vi "E441X_PM_Get_Sensor_Type.vi"(0 "VISA session":refnum<visa-resource-name>, 5 "Channel (0: A)":i32(ring) items=["A", "B"], 11 "error in (no error)":errorcluster {"code" format="%.0x"}) -> (4 "dup VISA session":refnum<visa-resource-name>, 6 "State":bool=TRUE, 10 "Sensor Type":string, 15 "error out":errorcluster {"code" format="%.0x"})   [LabVIEW 2015]
doc: "This VI returns the type of sensor connected to the selected input."
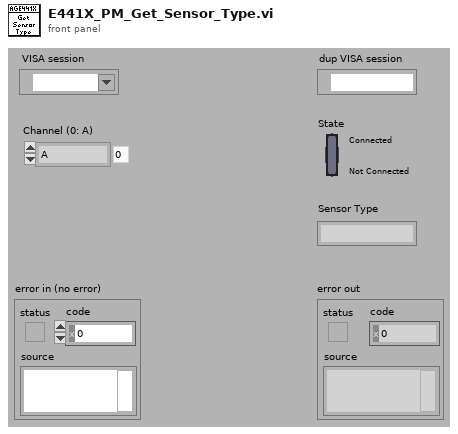
[diagram p1: front panel]
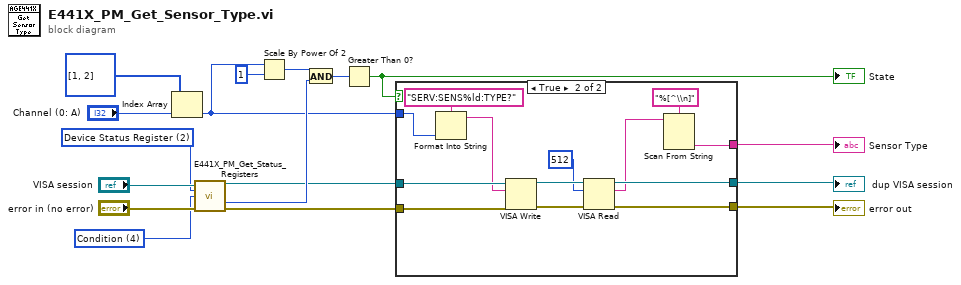
[diagram p0: block diagram]
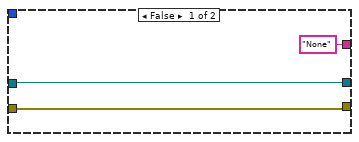
[diagram p2: hidden frame]
diagram:
  w14 = 4 items=["Enable"=2, "Negative Transition"=0, "Positive Transition"=1, "Event"=3, "Condition"=4] ("Register Part (2: Enable)")
  w15 = 2 items=["Service Request Enable Register (SRE)", "Standard Event Status Enable Register (ESE)", "Device Status Register", "Operation Status Register", "Questionable Status Register", "Operation Status Calibration", "Operation Status Measuring", "Operation Status Trigger", "Operation Status Sense", "Operation Status Low Limit Fail", "Operation Status Upper Limit Fail", "Questionable Status Power", "Questionable Status Calibration"] ("Register (4: Questionable Status Register)")
  n1 = Index Array(array=i32[] [1, 2], index="Channel (0: A)") -> (element=w1:i32)
  n2 = call "E441X_PM_Get_Status_Registers.vi"("VISA session"="VISA session", "Register (4: Questionable Status Register)"=w15, "Register Part (2: Enable)"=w14, "error in (no error)"="error in (no error)") -> ("dup VISA session"=w7:refnum<visa-resource-name>, "State"=w10:u16, "error out"=w6:errorcluster)  [unwired: 9 in]
  n3 = Scale By Power Of 2(n=w1, x=1) -> (x*2^n=w11:i32)
  n4 = And(x=w11, y=w10) -> (x .and. y?=w9:i32)
  n5 = Greater Than 0?(x=w9) -> (x > 0?=w8:bool)
  "State" <- w8
  n6 = case shown="True" w8 {
    tunnel: w7 -> [w19 w31]
    tunnel: w6 -> [w18 w30]
    tunnel: w1 -> [_ w32]
    tunnel: [w19 w25] -> w5
    tunnel: [w18 w24] -> w4
    tunnel: ["None" ("read buffer") w21] -> w3
    frame False {
    }
    frame True {
      n7 = Format Into String(format string="SERV:SENS%ld:TYPE?", w32) -> (resulting string=w29:string)  [unwired: 2 in, 1 out]
      n8 = VISA Write(VISA resource name=w31, write buffer=w29, error in (no error)=w30) -> (VISA resource name out=w28:refnum<visa-resource-name>, error out=w27:errorcluster)  [unwired: 1 out]
      n9 = VISA Read(VISA resource name=w28, byte count=u32 512 ("byte count (0)"), error in (no error)=w27) -> (VISA resource name out=w25:refnum<visa-resource-name>, read buffer=w22:string, error out=w24:errorcluster)  [unwired: 1 out]
      n10 = Scan From String(format string="%[^\\n]", input string=w22) -> (output 1=w21:string)  [unwired: 3 in, 3 out]
    }
  }
  "dup VISA session" <- w5
  "error out" <- w4
  "Sensor Type" <- w3
